vi "Read Measurement (RJDJ).vi"(0 "VISA resource name":refnum<visa-resource-name>, 5 "Maximum Time (10000ms)":u32, 11 "error in (no error)":errorcluster) -> (3 "TJ":T1, 4 "VISA resource name out":refnum<visa-resource-name>, 6 "DJ":T1, 8 "RJ":T1, 10 "PJ":T2, 12 "DDJ":T1, 13 "DCD":cluster{"Result":dbl, "State":i32}, 14 "ISI":T1, 15 "error out":errorcluster)   [LabVIEW 2009, in "Agilent 8000 Series.lvlib"]
doc: "Reads all the RDJD measurements. It initiates, waits for the acquisition to finish and returns the results of the RJDJ measurement."
uses:
  Agilent 8000 Series.lvlib
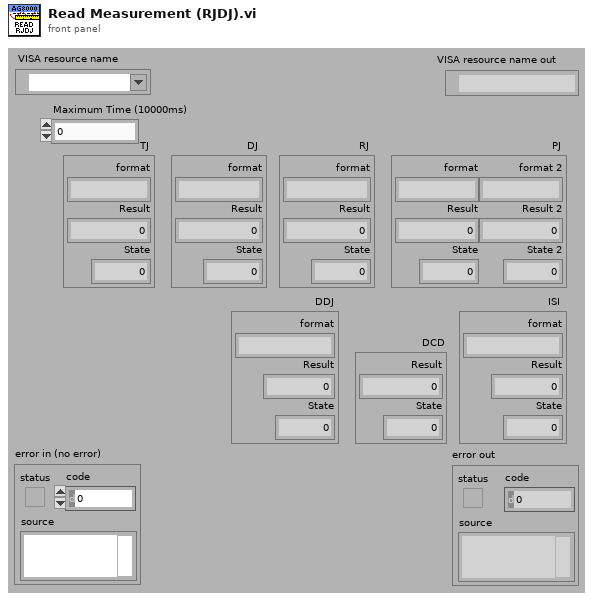
[diagram p1: front panel]
types:
  T1 = cluster{"format":string, "Result":dbl, "State":i32}
  T2 = cluster{"format":string, "Result":dbl, "State":i32, "format 2":string, "Result 2":dbl, "State 2":i32}
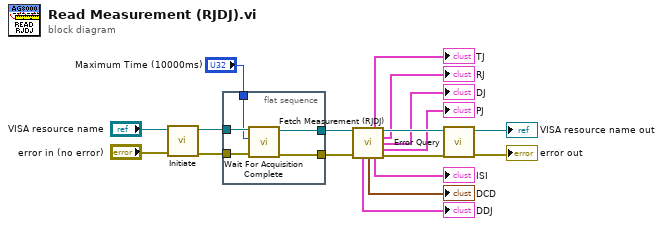
[diagram p0: block diagram]
diagram:
  n1 = call "Initiate.vi"("error in (no error)"="error in (no error)", "VISA resource name"="VISA resource name") -> ("error out"=w15:errorcluster, "VISA resource name out"=w16:refnum<visa-resource-name>)  [unwired: 8 in]
  n2 = flat-sequence {
    tunnel: w16 -> [w23]
    tunnel: w15 -> [w22]
    tunnel: [w21] -> w11
    tunnel: [w20] -> w10
    tunnel: "Maximum Time (10000ms)" -> [w19]
    frame #0 {
      n3 = call "Wait For Acquisition Complete.vi"("error in (no error)"=w22, "Maximum Time (10000ms)"=w19, "VISA resource name"=w23) -> ("error out"=w20:errorcluster, "VISA resource name out"=w21:refnum<visa-resource-name>)  [unwired: 7 in]
    }
  }
  n4 = call "Fetch Measurement (RJDJ).vi"("VISA resource name"=w11, "error in (no error)"=w10) -> ("TJ"=→"TJ":T1, "VISA resource name out"=w9:refnum<visa-resource-name>, "RJ"=→"RJ":T1, "DJ"=→"DJ":T1, "PJ"=→"PJ":T2, "DDJ"=→"DDJ":T1, "DCD"=→"DCD":cluster{"Result":dbl, "State":i32}, "ISI"=→"ISI":T1, "error out"=w8:errorcluster)  [unwired: 5 in]
  n5 = call "Error Query.vi"("error in (no error)"=w8, "VISA resource name"=w9) -> ("error out"=→"error out":errorcluster, "VISA resource name out"=→"VISA resource name out":refnum<visa-resource-name>)  [unwired: 6 in, 2 out]
